vi "VIA Minify all VIs.vi"(11 "VIA in":string) -> (2 "Bytes Removed":i32, 3 "VIA out":string)   [LabVIEW 2020]
uses:
  <vilib>/regexp/Match Regular Expression.xnode
panel:
  out "VI names":string[](array[string])
  out "Number of VIs Processed":i32
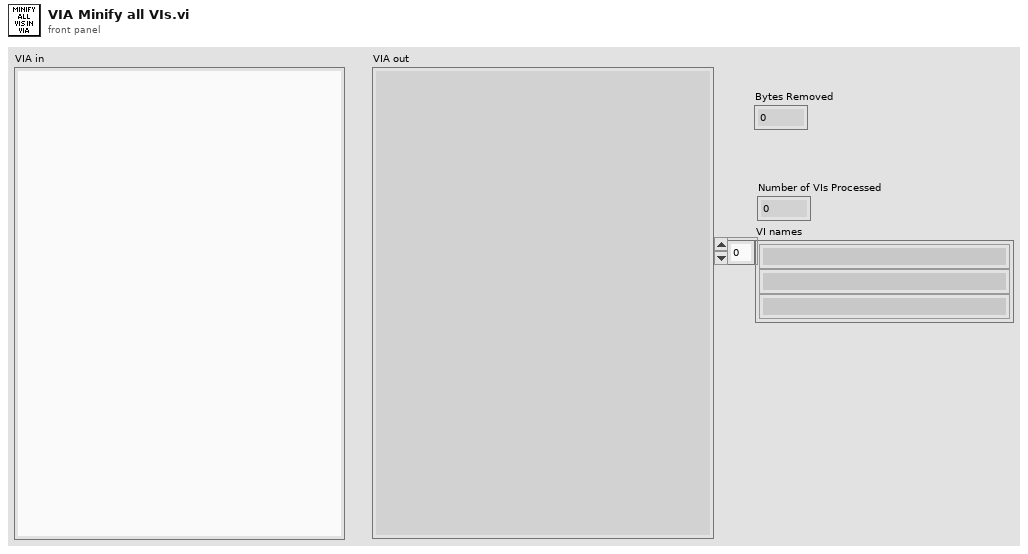
[diagram p1: front panel]
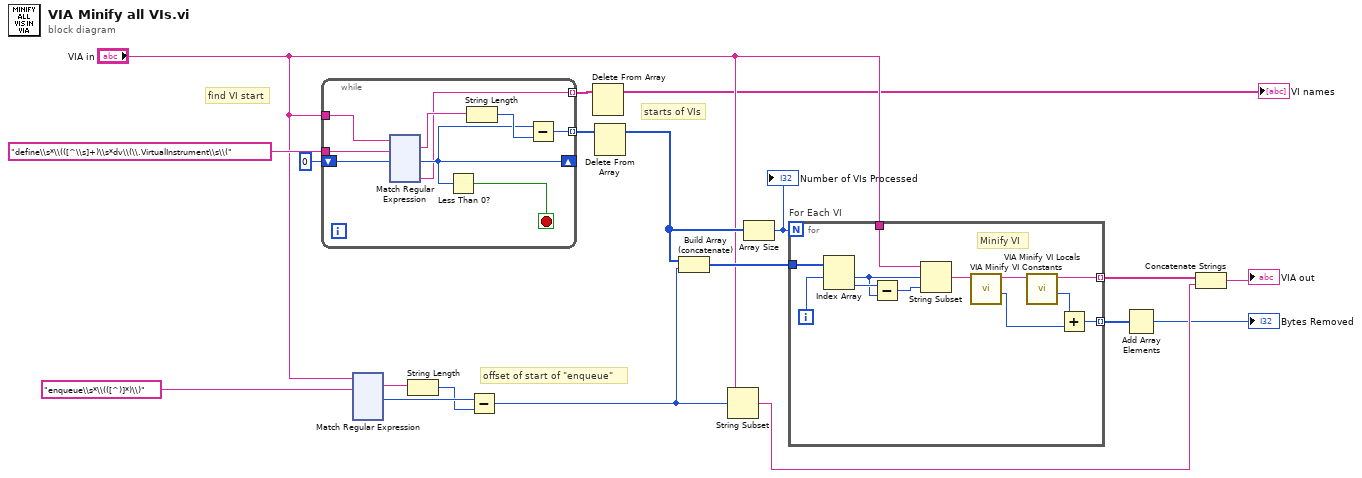
[diagram p0: block diagram]
diagram:
  # "starts of VIs"
  # "offset of start of \"enqueue\""
  # "find VI start"
  n1 = while {
    tunnel: "VIA in" -> [w28]
    tunnel: "define\\s*\\(([^\\s]+)\\s*dv\\(\\.VirtualInstrument\\s\\(" ("regular expression") -> [w27]
    shift-right: [w22] -> _
    shift-left: 0 ("offset (0)") -> [w26]
    tunnel: [w23] -> w13 mode=indexing
    tunnel: [w20] -> w2 mode=indexing
    stop <- w21 stop-if-true
    n2 = xnode "Match Regular Expression"("input string"=w28, "regular expression"=w27, "offset (0)"=w26) -> ("whole match"=w24:string, "offset past match"=w22:i32, "submatch 1"=w20:string)  [unwired: 3 in, 3 out]
    n3 = Less Than 0?(x=w22) -> (x < 0?=w21:bool)
    n4 = String Length(string=w24) -> (length=w25:i32)
    n5 = Subtract(x=w22, y=w25) -> (x-y=w23:i32)
  }
  n6 = xnode "Match Regular Expression"("input string"="VIA in", "regular expression"="enqueue\\s*\\(([^)]*)\\)") -> ("whole match"=w18:string, "offset past match"=w17:i32)  [unwired: 4 in, 4 out]
  n7 = String Length(string=w18) -> (length=w16:i32)
  n8 = Subtract(x=w17, y=w16) -> (x-y=w7:i32)
  n9 = Delete From Array(array=w2) -> (array with subset deleted=→"VI names":string[])  [unwired: 2 in, 1 out]
  n10 = Delete From Array(array=w13) -> (array with subset deleted=w10:i32[])  [unwired: 2 in, 1 out]
  n11 = Build Array (concatenate)(w10, w7) -> (w12:i32[])
  n12 = String Subset(string="VIA in", offset (0)=w7) -> (substring=w6:string)  [unwired: 1 in]
  n13 = Array Size(array=w10) -> (size(s)=w11:i32)
  "Number of VIs Processed" <- w11
  n14 = for "For Each VI" {
    N: w11 -> [_]
    tunnel: w12 -> [w156]
    tunnel: "VIA in" -> [w151]
    tunnel: [w146] -> w9 mode=indexing
    tunnel: [w145] -> w8 mode=indexing
    i -> [w155]
    # "Minify VI"
    n15 = Index Array(array=w156, index #1=w155) -> (element #1=w152:i32, element #2=w154:i32)  [unwired: 1 in]
    n16 = Subtract(x=w154, y=w152) -> (x-y=w153:i32)
    n17 = String Subset(string=w151, offset (0)=w152, length (rest)=w153) -> (substring=w147:string)
    n18 = call "VIA Minify VI Constants.vi"("VIA in"=w147) -> ("Bytes Removes"=w148:i32, "VIA out"=w150:string)  [unwired: 9 in]
    n19 = call "VIA Minify VI Locals.vi"("VIA in"=w150) -> ("Bytes Removes"=w149:i32, "VIA out"=w145:string)  [unwired: 8 in, 1 out]
    n20 = Add(x=w149, y=w148) -> (x+y=w146:i32)
  }
  n21 = Add Array Elements(numeric array=w9) -> (sum=→"Bytes Removed":i32)
  n22 = Concatenate Strings(w8, w6) -> (→"VIA out":string)
